vi "Last Ack Creator.vi"(10 "jettl":refnum<class "jettl.lvclass">, 11 "Base Event in":refnum<class "Base Event.lvclass">) -> (3 "Base Event out":refnum<class "Base Event.lvclass">)   [LabVIEW 2021, in "jettl.lvlib" / "Base Event.lvlib" / "Base Event.lvclass"]
uses:
  Base Event.lvclass
  Base Event.lvclass/Base Event.ctl
  jettl/jettl.lvclass
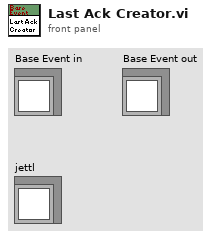
[diagram p1: front panel]
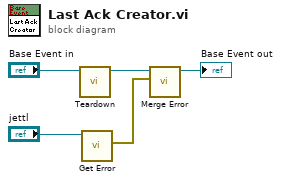
[diagram p0: block diagram]
diagram:
  n1 = call-dynamic "Teardown.vi"("Base Event in"="Base Event in") -> ("Base Event out"=w4:refnum<class "Base Event.lvclass">)  [unwired: 10 in]
  n2 = call-dynamic "Get Error.vi"("jettl in"="jettl") -> ("Error"=w5:errorcluster)  [unwired: 10 in]
  n3 = call-dynamic "Merge Error.vi"("Error"=w5, "Base Event in"=w4) -> ("Base Event out"=→"Base Event out":refnum<class "Base Event.lvclass">)  [unwired: 9 in]
